vi "Car_Speed_R567B.vi"(10 "精度":dbl=0.0625, 11 "车速":u16) -> (3 "报文":T1 {"[7]" format="%02x"; "[6]" format="%02x"; "[5]" format="%02x"; "[4]" format="%02x"; "[3]" format="%02x"; "[2]" format="%02x"; "[1]" format="%02x"; "[0]" format="%02x"})   [LabVIEW 2020]
uses:
  Global_Variable/Global.vi
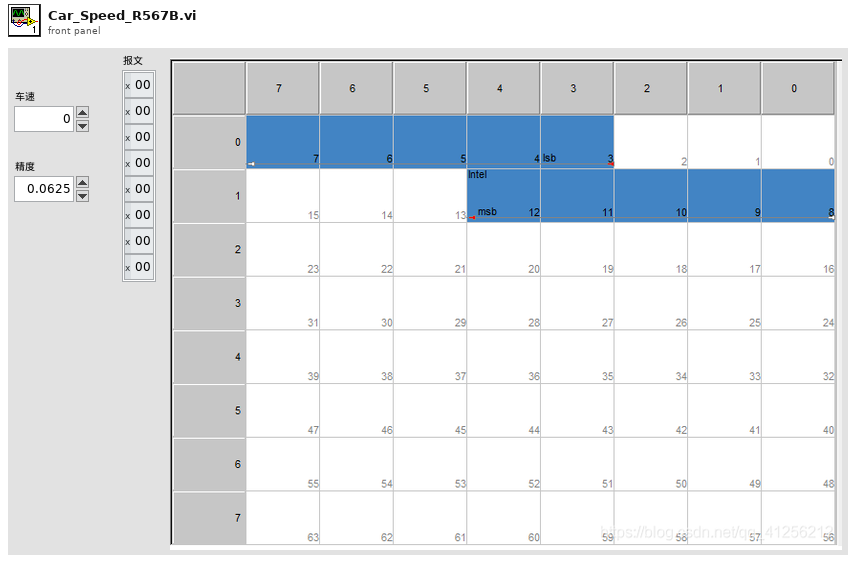
[diagram p1: front panel]
types:
  T1 = cluster{"[0]":u8, "[1]":u8, "[2]":u8, "[3]":u8, "[4]":u8, "[5]":u8, "[6]":u8, "[7]":u8}
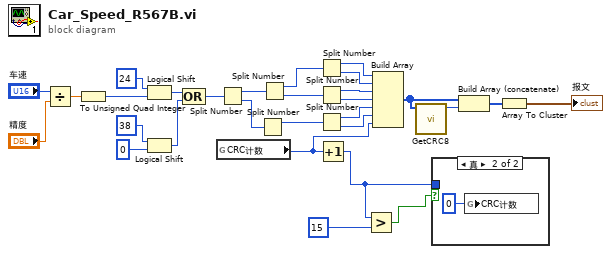
[diagram p0: block diagram]
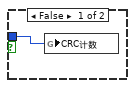
[diagram p2: hidden frame]
diagram:
  n1 = Divide(x="车速", y="精度") -> (x/y=w6:dbl)
  n2 = To Unsigned Quad Integer(1:w6) -> (0:w7:u64)
  n3 = Logical Shift(y=i16 24, x=w7) -> (x << y=w18:u64)
  n4 = Logical Shift(y=i16 38, x=u64 0) -> (x << y=w20:u64)
  n5 = Compound Arithmetic op=OR ("复合运算")(w18, w20) -> (w17:u64)
  n6 = global read "Global.vi" "CRC计数"() -> (w4:u8)
  n7 = Split Number(x=w17) -> (hi(x)=w26:u32, lo(x)=w25:u32)
  n8 = Split Number(x=w25) -> (hi(x)=w22:u16)  [unwired: 1 out]
  n9 = Split Number(x=w26) -> (hi(x)=w24:u16, lo(x)=w23:u16)
  n10 = Split Number(x=w24) -> (hi(x)=w16:u8, lo(x)=w15:u8)
  n11 = Split Number(x=w23) -> (hi(x)=w14:u8, lo(x)=w13:u8)
  n12 = Split Number(x=w22) -> (hi(x)=w12:u8, lo(x)=w11:u8)
  n13 = Increment(x=w4) -> (x+1=w1:u8)
  n14 = Greater?(x=w1, y=u8 15) -> (0:w2:bool)
  n15 = Build Array(w16, w15, w14, w13, w12, w11, w4) -> (w10:u8[])
  n16 = call "GetCRC8.vi"("xData"=w10) -> ("CRC8"=w9:u8)  [unwired: 9 in, 1 out]
  n17 = case shown="真" w2 {
    tunnel: w1 -> [w30 _]
    frame False {
      n18 = global write "Global.vi" "CRC计数"(w30) -> ()
    }
    frame True {
      n19 = global write "Global.vi" "CRC计数"(u8 0 ("CRC计数")) -> ()
    }
  }
  n20 = Build Array (concatenate)(w10, w9) -> (w8:u8[])
  n21 = Array To Cluster(array=w8) -> (cluster=→"报文":T1)
